vi "CSM - Start Async Call.vi"   [LabVIEW 2017, in "CSM-QuickDrops.lvlib"]
doc: "Code snippet for starting a CSM module asynchronously. After dragging this VI to the block diagram, change the static VI reference to the target CSM module.\n\nReference Example: `[CSM-Example]\\3. Caller is Other Framework Scenario\\CSM Example - Caller is NOT a CSM.vi`."
uses:
  CSM-QuickDrops.lvlib
  Communicable State Machine.lvlib
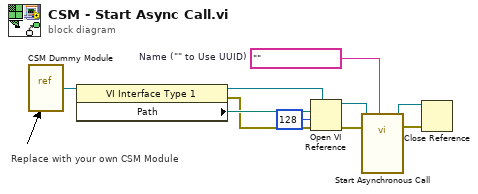
[diagram p0: block diagram]
diagram:
  w4 = ""  # Name ("" to Use UUID)
  # "Replace with your own CSM Module"
  n1 = vi-ref "CSM Dummy Module.vi"() -> (w9:refnum<vi>)
  n2 = property class="VI Interface Type 1"(reference=w9) -> (reference out=w5:refnum<vi>, error out=w7:errorcluster, "Path"=w8:path)  [unwired: 1 in]
  n3 = Open VI Reference(type specifier VI Refnum (for type only)=w5, vi path=w8, options=128, error in (no error)=w7) -> (vi reference=w6:refnum<vi>, error out=w10:errorcluster)  [unwired: 2 in]
  n4 = call-by-ref "Start Asynchronous Call"(reference=w6, error in=w10, "Name(\"\" to use uuid)"=w4) -> (reference out=w2:refnum<vi>, error out=w3:errorcluster)  [unwired: 11 in]
  n5 = Close Reference(reference=w2, error in (no error)=w3) -> ()  [unwired: 1 out]
